vi "DidYouJustPressButton1.vi"(6 "New Button Info":T1, 7 "Old Button Info":T1) -> (1 "Button1 Old State":bool, 2 "Button1 New State":bool, 3 "Did You Just Press Button1?":bool)   [LabVIEW 2014]
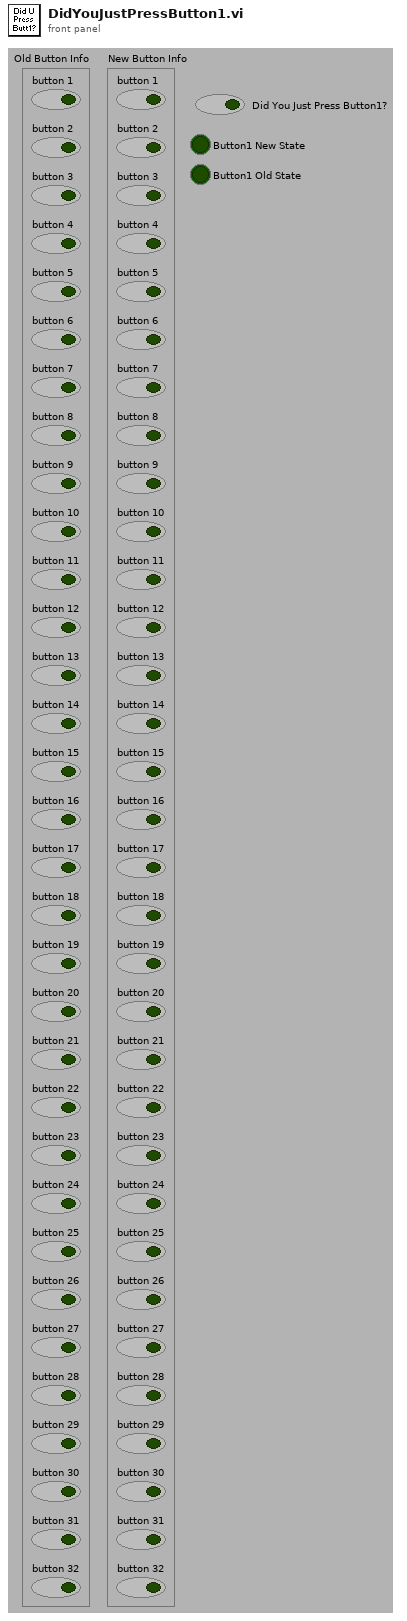
[diagram p1: front panel]
types:
  T1 = cluster{"button 1":bool, "button 2":bool, "button 3":bool, "button 4":bool, "button 5":bool, "button 6":bool, "button 7":bool, "button 8":bool, "button 9":bool, "button 10":bool, "button 11":bool, "button 12":bool, "button 13":bool, "button 14":bool, "button 15":bool, "button 16":bool, "button 17":bool, "button 18":bool, "button 19":bool, "button 20":bool, "button 21":bool, "button 22":bool, "button 23":bool, "button 24":bool, "button 25":bool, "button 26":bool, "button 27":bool, "button 28":bool, "button 29":bool, "button 30":bool, "button 31":bool, "button 32":bool}
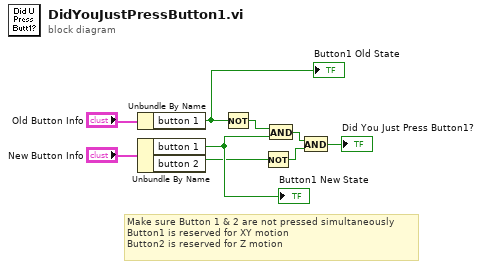
[diagram p0: block diagram]
diagram:
  # "Make sure Button 1 & 2 are not pressed simultaneously\nButton1 is reserved for XY motion\nButton2 is reserved for Z motion"
  n1 = Unbundle By Name("Old Button Info") -> ("button 1"=w7:bool)
  "Button1 Old State" <- w7
  n2 = Unbundle By Name("New Button Info") -> ("button 1"=w9:bool, "button 2"=w1:bool)
  "Button1 New State" <- w9
  n3 = Not(x=w7) -> (.not. x?=w8:bool)
  n4 = Not(x=w1) -> (.not. x?=w3:bool)
  n5 = And(x=w8, y=w9) -> (x .and. y?=w4:bool)
  n6 = And(x=w4, y=w3) -> (x .and. y?=→"Did You Just Press Button1?":bool)
